vi "get channels test.vi"() -> (0 "error out":errorcluster, 2 "channels match":bool)   [LabVIEW 2013, in "J1939 tests.lvlib"]
doc: "Tests the 'Get Channels' VI of the Configuration class."
uses:
  J1939 tests.lvlib
  module/configuration/J1939 configuration.lvclass
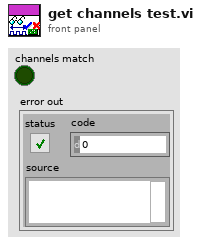
[diagram p1: front panel]
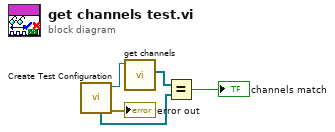
[diagram p0: block diagram]
diagram:
  n1 = call "Create Test Configuration.vi"() -> ("error out"=→"error out":errorcluster, "Module Configuration"=w3:refnum<class "J1939 configuration.lvclass">, "Channels"=w1:refnum<class "TBM channel.lvclass">[])  [unwired: 5 in, 4 out]
  n2 = call-dynamic "get channels.vi"("J1939 configuration in"=w3) -> ("channels"=w5:refnum<class "TBM channel.lvclass">[])  [unwired: 9 in, 1 out]
  n3 = Equal?(x=w5, y=w1) -> (x = y?=→"channels match":bool)
